vi "ClawExecute.vi"   [LabVIEW 2020]
uses:
  <vilib>/Rock Robotics/WPI/Solenoid/WPI_SolenoidValue.ctl
  <vilib>/Rock Robotics/WPI/Solenoid/WPI_SolenoidSetEnum.vi
types:
  T1 = typedef "WPI_SolenoidValue.ctl" = enum16{"Off", "On", "Forward", "Reverse"}
  T2 = typedef "WPI_SolenoidDevRef.ctl" = cluster{"DevStatus":errorcluster, "Pneumatics Control Module":u8, "Forward Solenoid Channel":T3, "Reverse Solenoid Channel":T3}
  T3 = typedef "WPI_SolenoidChannel.ctl" = enum8{"Solenoid 0", "Solenoid 1", "Solenoid 2", "Solenoid 3", "Solenoid 4", "Solenoid 5", "Solenoid 6", "Solenoid 7", "Solenoid 8", "Solenoid 9", "Solenoid 10", "Solenoid 11", "Solenoid 12", "Solenoid 13", "Solenoid 14", "Solenoid 15", "Invalid"}
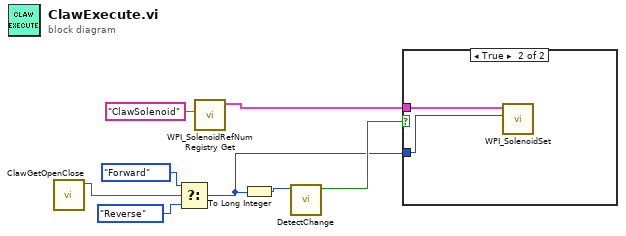
[diagram p0: block diagram]
diagram:
  n1 = call "ClawGetOpenClose.vi"() -> ("Open?"=w7:bool)  [unwired: 11 in]
  n2 = Select(t=WPI_SolenoidValue."Forward" ("Value"), s=w7, f=WPI_SolenoidValue."Reverse" ("Value")) -> (s? t:f=w2:T1)
  n3 = call <vilib>:"WPI_SolenoidRefNum Registry Get.vi"("refnum name"="ClawSolenoid") -> ("SolenoidDevRef"=w4:T2)  [unwired: 9 in, 1 out]
  n4 = To Long Integer(number=w2) -> (32bit integer=w1:i32)
  n5 = call "DetectChange.vi"("Value"=w1) -> ("Changed"=w3:bool)  [unwired: 10 in]
  n6 = case shown="True" w3 {
    tunnel: w4 -> [_ w10]
    tunnel: w2 -> [_ w9]
    frame False {
    }
    frame True {
      n7 = call-poly <vilib>:"WPI_SolenoidSet.vi"("Value"=w9, "SolenoidDevRef"=w10) -> ()  [unwired: 8 in, 2 out]
    }
  }
